vi "setFPGAReference.vi"(10 "FPGAReference":refnum<k20>, 11 "FPGA in":refnum<class "FPGA.lvclass">) -> (3 "FPGA out":refnum<class "FPGA.lvclass">)   [LabVIEW 2016, in "FPGA.lvclass"]
uses:
  FPGA.lvclass
  FPGA.lvclass/FPGA.ctl
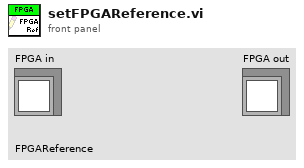
[diagram p1: front panel]
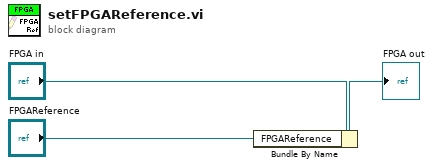
[diagram p0: block diagram]
diagram:
  n1 = Bundle By Name(cluster="FPGA in", "FPGAReference"="FPGAReference") -> (→"FPGA out":refnum<class "FPGA.lvclass">)
